vi "NIDMM_ReadDMM.vi"(7 "Measure Type":T1, 8 "error in (no error)":errorcluster, 9 "Range":dbl=-1.0, 10 "Resolution":T2=5.5 items=["3 1/2"=3.5, "4 1/2"=4.5, "5 1/2"=5.5, "6 1/2"=6.5, "7 1/2"=7.5], 11 "instrument handle":refnum<k15>) -> (0 "error out":errorcluster, 2 "Measurement":dbl)   [LabVIEW 2015]
uses:
  <instrlib>/niDMM/nidmm.llb/niDMM Resolution in Digits.ctl
  <instrlib>/niDMM/nidmm.llb/niDMM Function.ctl
  <instrlib>/niDMM/nidmm.llb/niDMM Configure Measurement Digits.vi
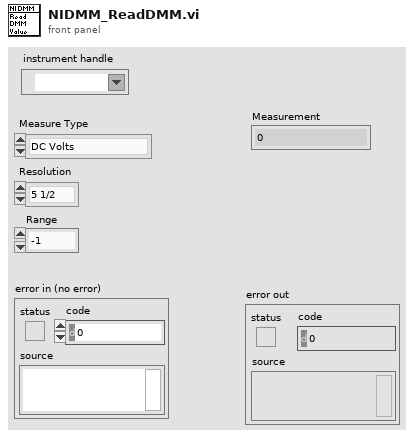
[diagram p1: front panel]
types:
  T1 = typedef "niDMM Function.ctl" = enum16{"DC Volts", "AC Volts", "DC Current", "AC Current", "2-wire Resistance", "4-wire Resistance", "Diode", "Frequency", "Period", "AC Volts DC Coupled", "Capacitance", "Inductance", "Temperature"}
  T2 = typedef "niDMM Resolution in Digits.ctl" = dbl
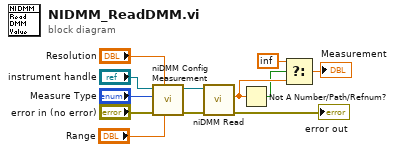
[diagram p0: block diagram]
diagram:
  n1 = call-poly <instrlib>:"niDMM Config Measurement.vi"("Range"="Range", "Resolution in Digits"="Resolution", "error in (no error)"="error in (no error)", "Function"="Measure Type", "instrument handle"="instrument handle") -> ("error out"=w12:errorcluster, "instrument handle out"=w10:refnum<k15>)  [unwired: 5 in]
  n2 = call <instrlib>:"niDMM Read.vi"("error in (no error)"=w12, "instrument handle"=w10) -> ("error out"=→"error out":errorcluster, "Measurement"=w8:dbl)  [unwired: 7 in, 1 out]
  n3 = Not A Number/Path/Refnum?(number/path/refnum=w8) -> (NaN/Path/Refnum?=w7:bool)
  n4 = Select(t=inf, s=w7, f=w8) -> (s? t:f=→"Measurement":dbl)
